vi "Lab.09_BP.vi"() -> ()   [LabVIEW 2016]
uses:
  <vilib>/Analysis/2dsp.llb/Real FFT.vi
  <vilib>/Analysis/baseanly.llb/Mean (DBL).vi
  <vilib>/Analysis/NI_AAL_SigProc.lvlib
  <vilib>/Analysis/NI_AALPro.lvlib
  <vilib>/Analysis/NI_AALBase.lvlib
panel:
  out "Pressure":dbl
  out "MIC_threshold":dbl
  out "freq_threshold":dbl
  out "pulse":dbl
  out "State":string
  out "Frequency analysis":dbl(graph)
  out "Status":string
  out "pulse LED":bool
  out "LBP":bool
  out "HBP":bool
  out "Pressure amp":dbl
  out "DIA":dbl=inf
  out "SYS":dbl=-inf caption="max"
  out "MIC amp":dbl
  out "MIC":dynamicdata(graph)
  out "Pressure signal":dynamicdata(graph)
  in  "stop":bool
  # "sphygmomanometer"
  # "mmHg"
  # "mmHg"
  # "/min"
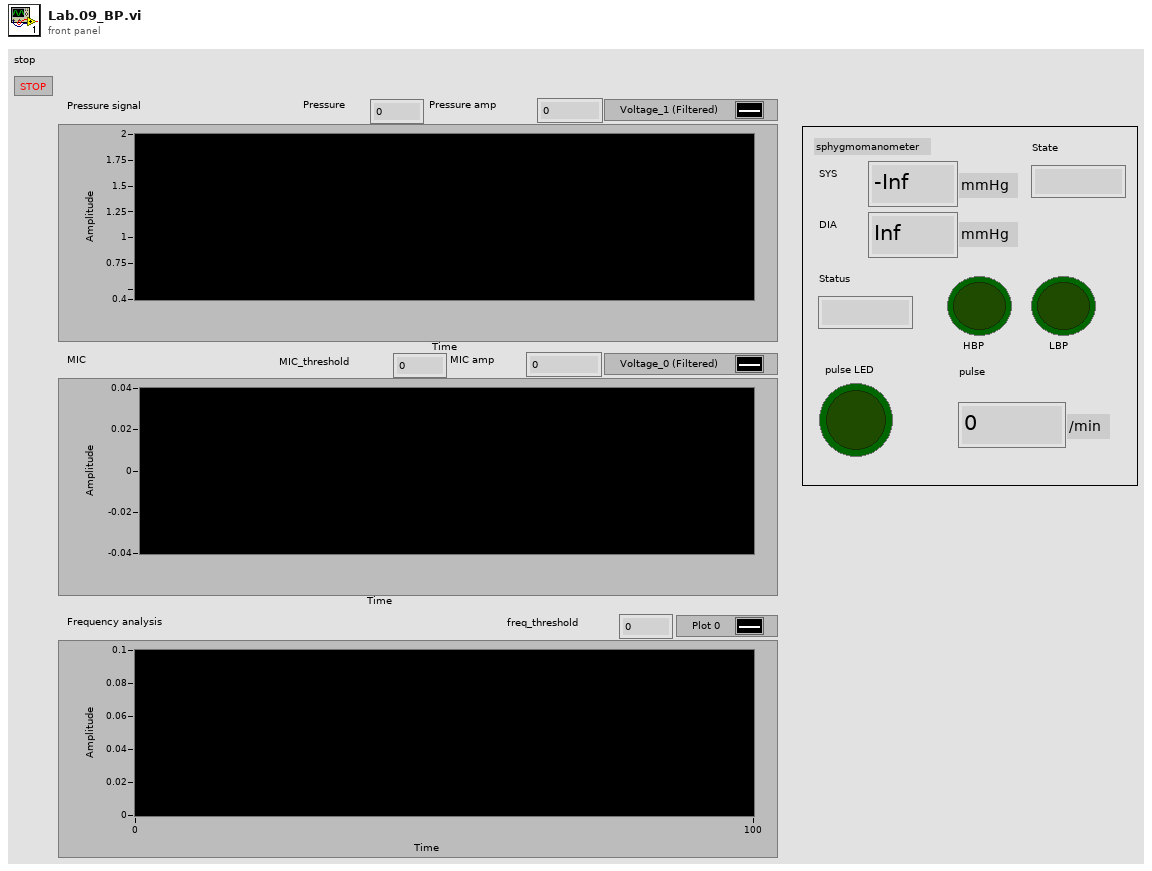
[diagram p1: front panel]
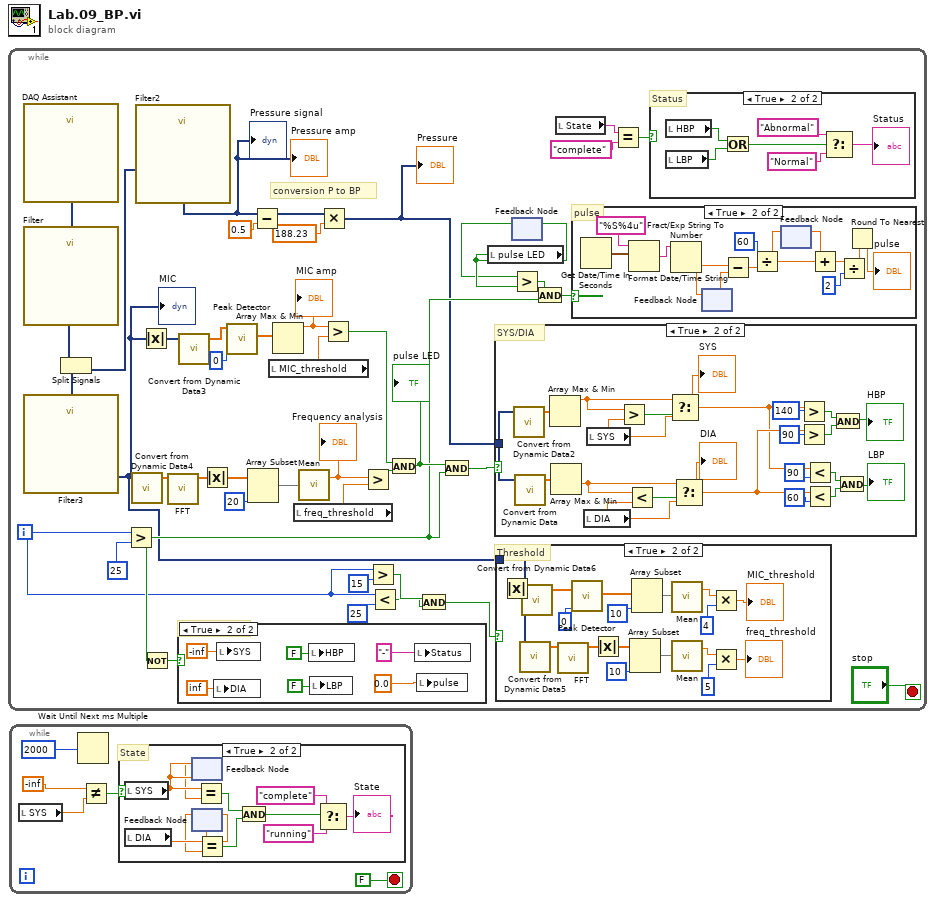
[diagram p0: block diagram]
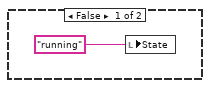
[diagram p2: hidden frame]
diagram:
  n1 = while {
    i -> [w6]
    stop <- "stop" stop-if-true
    # "Status"
    # "conversion P to BP"
    # "pulse"
    # "SYS/DIA"
    # "Threshold"
    # "default value"
    n2 = call "DAQ Assistant"() -> ("data"=w36:dynamicdata)  [unwired: 16 in, 3 out]
    n3 = call "Filter"("Signal"=w36) -> ("Filtered Signal"=w43:dynamicdata)  [unwired: 9 in, 1 out]
    n4 = Split Signals(w43) -> (w34:dynamicdata, w44:dynamicdata)  [unwired: 2 in]
    n5 = call "Filter3"("Signal"=w34) -> ("Filtered Signal"=w7:dynamicdata)  [unwired: 9 in, 1 out]
    "MIC" <- w7
    n6 = Greater?(x=w6, y=25) -> (0:w14:bool)
    n7 = call "Convert from Dynamic Data4"("Dynamic Data Type"=w7) -> ("Array"=w30:dbl[])  [unwired: 3 in]
    n8 = call "Filter2"("Signal"=w44) -> ("Filtered Signal"=w40:dynamicdata)  [unwired: 9 in, 1 out]
    "Pressure signal" <- w40
    "Pressure amp" <- w40
    n9 = Absolute Value(x=w7) -> (abs(x)=w26:dynamicdata)
    n10 = Not(x=w14) -> (.not. x?=w37:bool)
    n11 = call-poly <vilib>:"FFT.vi"("X"=w30) -> ("FFT {X}"=w33:cdb[])  [unwired: 9 in, 1 out]
    n12 = case shown="True" w37 {
      frame False {
      }
      frame True {
        n13 = local write "DIA"(inf) -> ()
        n14 = local write "SYS"(-inf) -> ()
        n15 = local write "HBP"(FALSE) -> ()
        n16 = local write "LBP"(FALSE) -> ()
        n17 = local write "Status"("-") -> ()
        n18 = local write "pulse"(0.0) -> ()
      }
    }
    n19 = call "Convert from Dynamic Data3"("Dynamic Data Type"=w26) -> ("Array"=w25:dbl[])  [unwired: 3 in]
    n20 = Absolute Value(x=w33) -> (abs(x)=w29:dbl[])
    n21 = call <vilib>:"Peak Detector.vi"("peaks/valleys"=0, "X"=w25) -> ("Amplitudes"=w24:dbl[])  [unwired: 5 in, 4 out]
    n22 = Array Subset(array=w29, length=20) -> (w31:dbl[])  [unwired: 1 in]
    n23 = Subtract(x=w40, y=0.5) -> (x-y=w38:dynamicdata)
    n24 = local read "MIC_threshold"() -> (w19:dbl)
    n25 = Array Max & Min(array=w24) -> (max value=w1:dbl)  [unwired: 3 out]
    "MIC amp" <- w1
    n26 = local read "freq_threshold"() -> (w13:dbl)
    n27 = call-poly <vilib>:"Mean.vi"("X"=w31) -> ("mean"=w28:dbl)  [unwired: 1 out]
    "Frequency analysis" <- w28
    n28 = Multiply(x=w38, y=188.23) -> (x*y=w2:dynamicdata)
    "Pressure" <- w2
    n29 = Greater?(x=w1, y=w19) -> (0:w22:bool)
    n30 = Greater?(x=w28, y=w13) -> (0:w23:bool)
    n31 = Greater?(x=w6, y=15) -> (0:w10:bool)
    n32 = Less?(x=w6, y=25) -> (x < y?=w9:bool)
    n33 = And(x=w22, y=w23) -> (x .and. y?=w21:bool)
    "pulse LED" <- w21
    n34 = And(x=w10, y=w9) -> (x .and. y?=w8:bool)
    n35 = And(x=w21, y=w14) -> (x .and. y?=w20:bool)
    n36 = local read "pulse LED"() -> (w18:bool)
    n37 = case shown="True" w20 {
      tunnel: w2 -> [_ w101]
      frame False {
      }
      frame True {
        n38 = call "Convert from Dynamic Data2"("Dynamic Data Type"=w101) -> ("Array"=w102:dbl[])  [unwired: 3 in]
        n39 = call "Convert from Dynamic Data"("Dynamic Data Type"=w101) -> ("Array"=w103:dbl[])  [unwired: 3 in]
        n40 = Array Max & Min(array=w102) -> (max value=w107:dbl)  [unwired: 3 out]
        n41 = Array Max & Min(array=w103) -> (min value=w105:dbl)  [unwired: 3 out]
        n42 = local read "DIA"() -> (w88:dbl)
        n43 = local read "SYS"() -> (w104:dbl)
        n44 = Greater?(x=w107, y=w104) -> (0:w108:bool)
        n45 = Less?(x=w105, y=w88) -> (x < y?=w106:bool)
        n46 = Select(t=w107, s=w108, f=w104) -> (s? t:f=w89:dbl)
        "SYS" <- w89
        n47 = Select(t=w105, s=w106, f=w88) -> (s? t:f=w95:dbl)
        "DIA" <- w95
        n48 = Greater?(x=w89, y=140) -> (0:w98:bool)
        n49 = Greater?(x=w95, y=90) -> (0:w97:bool)
        n50 = Less?(x=w89, y=90) -> (x < y?=w92:bool)
        n51 = Less?(x=w95, y=60) -> (x < y?=w91:bool)
        n52 = And(x=w98, y=w97) -> (x .and. y?=→"HBP":bool)
        n53 = And(x=w92, y=w91) -> (x .and. y?=→"LBP":bool)
      }
    }
    n54 = case shown="True" w8 {
      tunnel: w7 -> [_ w59]
      frame False {
      }
      frame True {
        n55 = Absolute Value(x=w59) -> (abs(x)=w60:dynamicdata)
        n56 = call "Convert from Dynamic Data5"("Dynamic Data Type"=w59) -> ("Array"=w62:dbl[])  [unwired: 3 in]
        n57 = call "Convert from Dynamic Data6"("Dynamic Data Type"=w60) -> ("Array"=w58:dbl[])  [unwired: 3 in]
        n58 = call-poly <vilib>:"FFT.vi"("X"=w62) -> ("FFT {X}"=w63:cdb[])  [unwired: 9 in, 1 out]
        n59 = call <vilib>:"Peak Detector.vi"("peaks/valleys"=0, "X"=w58) -> ("Amplitudes"=w56:dbl[])  [unwired: 5 in, 4 out]
        n60 = Absolute Value(x=w63) -> (abs(x)=w66:dbl[])
        n61 = Array Subset(array=w66, length=10) -> (w65:dbl[])  [unwired: 1 in]
        n62 = Array Subset(array=w56, length=10) -> (w53:dbl[])  [unwired: 1 in]
        n63 = call-poly <vilib>:"Mean.vi"("X"=w53) -> ("mean"=w55:dbl)  [unwired: 1 out]
        n64 = call-poly <vilib>:"Mean.vi"("X"=w65) -> ("mean"=w67:dbl)  [unwired: 1 out]
        n65 = Multiply(x=w55, y=4) -> (x*y=→"MIC_threshold":dbl)
        n66 = Multiply(x=w67, y=5) -> (x*y=→"freq_threshold":dbl)
      }
    }
    n67 = feedback #1() -> (w17:bool)  [unwired: 1 in]
    n68 = feedback-in #1(w18) -> ()
    n69 = Greater?(x=w17, y=w18) -> (0:w16:bool)
    n70 = And(x=w16, y=w14) -> (x .and. y?=w15:bool)
    n71 = local read "State"() -> (w4:string)
    n72 = case shown="True" w15 {
      frame False {
      }
      frame True {
        n73 = Get Date/Time In Seconds() -> (seconds since 1Jan1904=w78:timestamp)
        n74 = Format Date/Time String(time format string (%c)="%S%4u", seconds (now)=w78) -> (date/time string=w79:string)  [unwired: 1 in]
        n75 = Fract/Exp String To Number(string=w79) -> (number=w81:dbl)  [unwired: 3 in, 1 out]
        n76 = feedback #2() -> (w80:dbl)  [unwired: 1 in]
        n77 = feedback-in #2(w81) -> ()
        n78 = Subtract(x=w81, y=w80) -> (x-y=w76:dbl)
        n79 = Divide(x=60, y=w76) -> (x/y=w73:dbl)
        n80 = feedback-in #3(w73) -> ()
        n81 = feedback #3() -> (w74:dbl)  [unwired: 1 in]
        n82 = Add(x=w74, y=w73) -> (x+y=w71:dbl)
        n83 = Divide(x=w71, y=2) -> (x/y=w70:dbl)
        n84 = Round To Nearest(number=w70) -> (nearest integer value=→"pulse":dbl)
      }
    }
    n85 = Equal?(x=w4, y="complete") -> (x = y?=w3:bool)
    n86 = case shown="True" w3 {
      frame False {
      }
      frame True {
        n87 = local read "HBP"() -> (w49:bool)
        n88 = local read "LBP"() -> (w48:bool)
        n89 = Or(x=w49, y=w48) -> (x .or. y?=w45:bool)
        n90 = Select(t="Abnormal", s=w45, f="Normal") -> (s? t:f=→"Status":string)
      }
    }
  }
  n91 = while {
    stop <- FALSE stop-if-true
    # "State"
    n92 = local read "SYS"() -> (w111:dbl)
    n93 = Wait Until Next ms Multiple(millisecond multiple=2000) -> ()  [unwired: 1 out]
    n94 = Not Equal?(x=-inf, y=w111) -> (x != y?=w110:bool)
    n95 = case shown="True" w110 {
      frame False {
        n96 = local write "State"("running") -> ()
      }
      frame True {
        n97 = local read "SYS"() -> (w122:dbl)
        n98 = local read "DIA"() -> (w116:dbl)
        n99 = feedback #4(w122) -> (w119:dbl)
        n100 = feedback-in #4(w122) -> ()
        n101 = feedback #5(w116) -> (w115:dbl)
        n102 = feedback-in #5(w116) -> ()
        n103 = Equal?(x=w122, y=w119) -> (x = y?=w120:bool)
        n104 = Equal?(x=w116, y=w115) -> (x = y?=w121:bool)
        n105 = And(x=w120, y=w121) -> (x .and. y?=w123:bool)
        n106 = Select(t="complete", s=w123, f="running") -> (s? t:f=→"State":string)
      }
    }
  }
